vi "Open Experiment VI.vi"(8 "error in (no error)":errorcluster, 11 "Path":path) -> (0 "error out":errorcluster)   [LabVIEW 2019, in "Control Experiment.lvclass"]
uses:
  <userlib>/LevyLab/Transport/Control Experiment/Control Experiment.lvclass
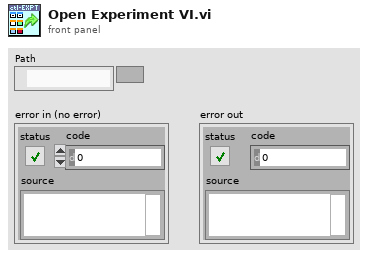
[diagram p1: front panel]
types:
  T1 = enum32{"Invalid", "Standard", "Closed", "Hidden", "Minimized", "Maximized"}
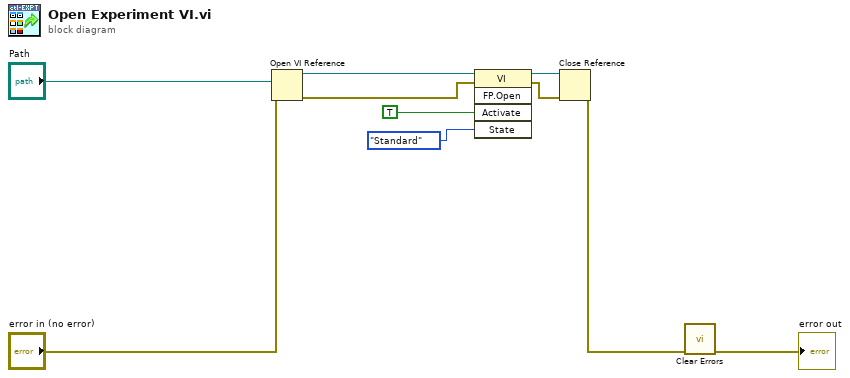
[diagram p0: block diagram]
diagram:
  n1 = Open VI Reference(vi path="Path", error in (no error)="error in (no error)") -> (vi reference=w7:refnum<vi>, error out=w2:errorcluster)  [unwired: 4 in]
  n2 = invoke class="VI" method="FP.Open"(reference=w7, error in=w2, "Activate"=TRUE ("Activate?"), "State"=T1."Standard") -> (reference out=w6:refnum<vi>, error out=w5:errorcluster)  [unwired: 1 in, 3 out]
  n3 = Close Reference(reference=w6, error in (no error)=w5) -> (error out=w9:errorcluster)
  n4 = call <vilib>:"Clear Errors.vi"("error in (no error)"=w9) -> ("error out"=→"error out":errorcluster)  [unwired: 5 in, 1 out]
